vi "Run Test (Array Path).vi"(5 "Test Report":refnum<class "Test Report.lvclass">, 6 "Verbose":bool, 7 "Report Path":path, 8 "error in":errorcluster, 9 "Inspect Recursively (T)":bool=TRUE, 10 "Paths":path[](array[path]), 11 "Interactive (T)":bool=TRUE) -> (0 "error out":errorcluster)   [LabVIEW 2013, in "Caraya.lvlib"]
uses:
  Caraya.lvlib
  classes/Test Report/Test Report.lvclass
  <userlib>/_OpenG.lib/file/file.llb/Valid Path - Array__ogtk.vi
  <userlib>/_OpenG.lib/file/file.llb/File Exists - Array__ogtk.vi
  classes/Test Runner/Test Runner.lvclass
  classes/Test Runner.Folder/Test Runner.Folder.lvclass
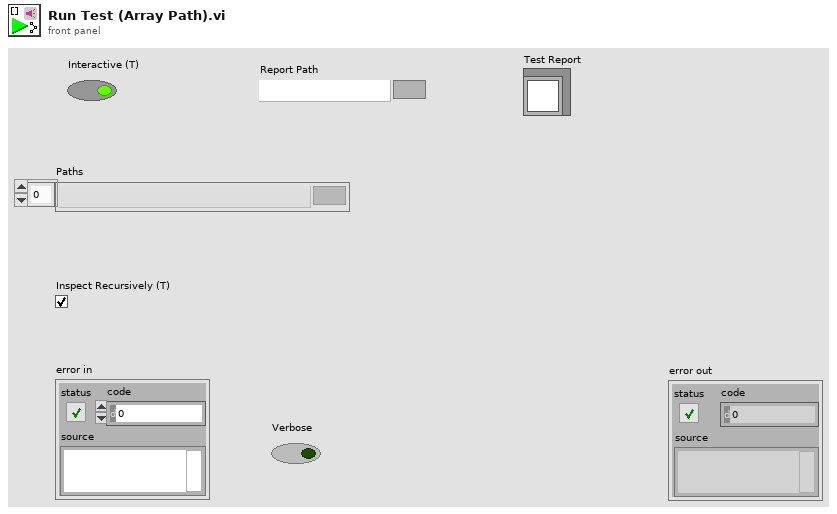
[diagram p1: front panel]
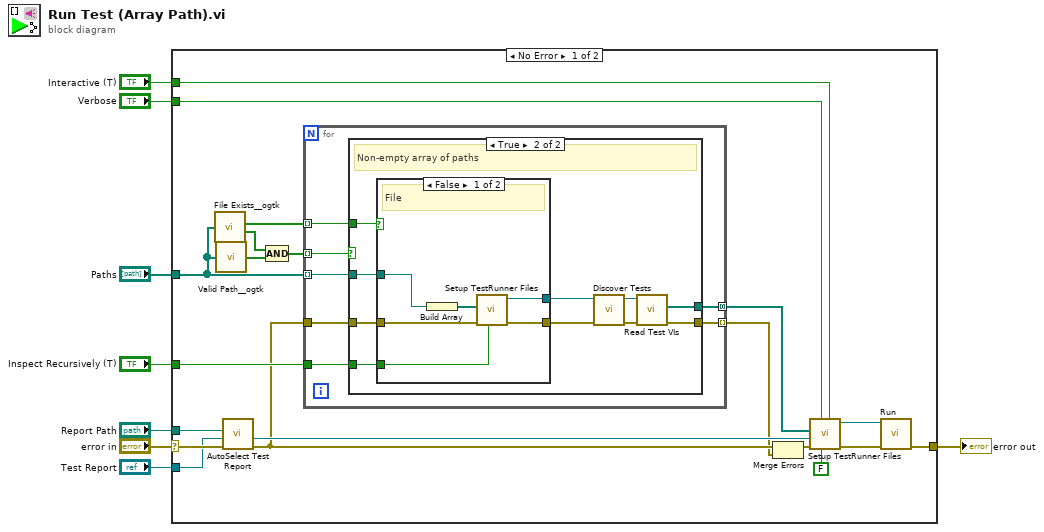
[diagram p0: block diagram]
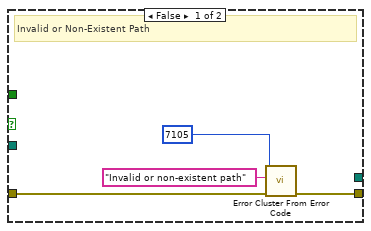
[diagram p2: hidden frame]
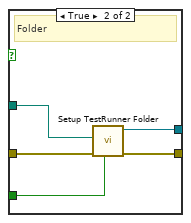
[diagram p3: hidden frame]
diagram:
  n1 = case shown="No Error" "error in" {
    selector: "error in" -> [w28 w61]
    tunnel: [w16 w61] -> w8
    tunnel: "Verbose" -> [w12 _]
    tunnel: "Interactive (T)" -> [w13 _]
    tunnel: "Test Report" -> [w26 _]
    tunnel: "Paths" -> [w24 _]
    tunnel: "Report Path" -> [w27 _]
    tunnel: "Inspect Recursively (T)" -> [w14 _]
    frame No Error {
      n2 = call-poly <userlib>:"File Exists__ogtk.vi"("file paths"=w24) -> ("is directory"=w21:bool[], "exists"=w25:bool[])  [unwired: 6 in]
      n3 = call-poly <userlib>:"Valid Path__ogtk.vi"("array of paths"=w24) -> ("valid"=w23:bool[])
      n4 = call "AutoSelect Test Report.vi"("error in (no error)"=w28, "Test Report in"=w26, "Report Path"=w27) -> ("error out"=w10:errorcluster, "Test Report out"=w15:refnum<class "Test Report.lvclass">)  [unwired: 7 in]
      n5 = Compound Arithmetic op=AND(w25, w23) -> (w22:bool[])
      n6 = for {
        tunnel: [w35] -> w9 mode=indexing
        tunnel: w10 -> [w34]
        tunnel: w14 -> [w33]
        tunnel: w24 -> [w32] mode=indexing
        tunnel: w22 -> [w31] mode=indexing
        tunnel: w21 -> [w30] mode=indexing
        tunnel: [w29] -> w20 mode=concatenating
        n7 = case shown="True" w31 {
          tunnel: [w38 w41] -> w35
          tunnel: w34 -> [w39 w49]
          tunnel: w33 -> [_ w48]
          tunnel: w32 -> [_ w47]
          tunnel: w30 -> [_ w46]
          tunnel: [_ w40] -> w29
          frame False {
            # "Invalid or Non-Existent Path"
            n8 = call <vilib>:"Error Cluster From Error Code.vi"("error in (no error)"=w39, "error message (\"\")"="Invalid or non-existent path" ("error message (\"\")"), "error code (0)"=7105 ("code")) -> ("error out"=w38:errorcluster)  [unwired: 6 in]
          }
          frame True {
            # "Non-empty array of paths"
            n9 = case shown="False" w46 {
              tunnel: [w54 w56] -> w43
              tunnel: [w53 w57] -> w44
              tunnel: w49 -> [w55 w60]
              tunnel: w47 -> [w52 w58]
              tunnel: w48 -> [w51 w59]
              frame False {
                # "File"
                n10 = Build Array(w52) -> (w50:path[])
                n11 = call "Setup TestRunner Files.vi"("Inspect Recursively (T)"=w51, "error in (no error)"=w55, "Paths"=w50) -> ("error out"=w54:errorcluster, "Test Runner.Folder out"=w53:refnum<class "Test Runner.Folder.lvclass">)  [unwired: 7 in]
              }
              frame True {
                # "Folder"
                n12 = call "Setup TestRunner Folder.vi"("Inspect Recursively (T)"=w59, "error in (no error)"=w60, "Directory to search"=w58) -> ("error out"=w56:errorcluster, "Test Runner.Folder out"=w57:refnum<class "Test Runner.Folder.lvclass">)  [unwired: 7 in]
              }
            }
            n13 = call "Discover Tests.vi"("error in (no error)"=w43, "Test Runner in"=w44) -> ("error out"=w42:errorcluster, "Test Runner out"=w45:refnum<class "Test Runner.Folder.lvclass">)  [unwired: 8 in]
            n14 = call "Read Test VIs.vi"("error in (no error)"=w42, "Test Runner in"=w45) -> ("error out"=w41:errorcluster, "Test VIs"=w40:path[])  [unwired: 7 in, 1 out]
          }
        }
      }
      n15 = Merge Errors(w10, w9) -> (w19:errorcluster)
      n16 = call "Setup TestRunner Files.vi"("Interactive (T)"=w13, "Inspect Recursively (T)"=FALSE, "Verbose (F)"=w12, "error in (no error)"=w19, "Test Report"=w15, "Paths"=w20) -> ("error out"=w17:errorcluster, "Test Runner.Folder out"=w18:refnum<class "Test Runner.Folder.lvclass">)  [unwired: 4 in]
      n17 = call "Run.vi"("error in (no error)"=w17, "Test Runner in"=w18) -> ("error out"=w16:errorcluster)  [unwired: 8 in, 1 out]
    }
    frame Error {
    }
  }
  "error out" <- w8
